vi "Check And Clear Missing Messages - XY Chart.vi"(9 "index":i32, 11 "AScan+Peaks in":cluster{"timebase":dbl[], "data":u16[]}[](array[cluster])) -> (1 "Running Average PRF":dbl, 3 "AScan+Peaks out":cluster{"timebase":dbl[], "data":u16[]}[](array[cluster]))   [LabVIEW 2026, in "MicroPulse_Driver.lvlib"]
uses:
  MicroPulse_Driver.lvlib
  <vilib>/ptbypt/NI_PtbyPt.lvlib
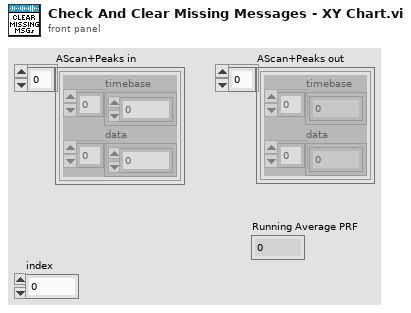
[diagram p1: front panel]
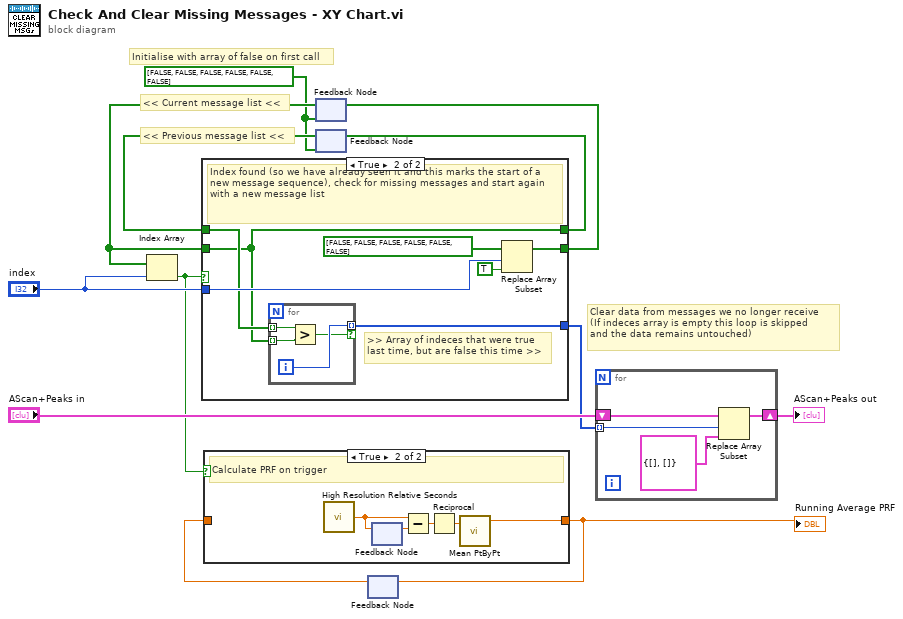
[diagram p0: block diagram]
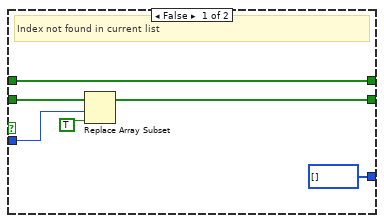
[diagram p3: hidden frame]
diagram:
  w7 = bool[] [FALSE, FALSE, FALSE, FALSE, FALSE, FALSE]
  # "Clear data from messages we no longer receive\n(If indeces array is empty this loop is skipped\nand the data remains untouched)"
  # "Initialise with array of false on first call"
  # "<< Previous message list <<"
  # "<< Current message list <<"
  n1 = feedback #1(w7) -> (w9:bool[])
  n2 = Index Array(array=w9, index="index") -> (element=w1:bool)
  n3 = feedback #2(w7) -> (w11:bool[])
  n4 = case shown="True" w1 {
    tunnel: "index" -> [w18 w23]
    tunnel: w9 -> [w17 w20]
    tunnel: [w16 w24] -> w12
    tunnel: w11 -> [w15 w21]
    tunnel: [w15 w20] -> w10
    tunnel: [i32[] [] w19] -> w5
    frame False {
      # "Index not found in current list"
      n5 = Replace Array Subset(array=w17, new element=TRUE, index=w18) -> (w16:bool[])
    }
    frame True {
      # ">> Array of indeces that were true\nlast time, but are false this time >>"
      # "Index found (so we have already seen it and this marks the start of a new message sequence), check for missing messages and start again with a new message list"
      n6 = for {
        tunnel: w21 -> [w29] mode=indexing
        tunnel: w20 -> [w28] mode=indexing
        tunnel: [w27] -> w19 mode=indexing if=w26
        i -> [w27]
        n7 = Greater?(x=w29, y=w28) -> (0:w26:bool)
      }
      n8 = Replace Array Subset(array=bool[] [FALSE, FALSE, FALSE, FALSE, FALSE, FALSE], new element=TRUE ("new element/subarray"), index=w23) -> (w24:bool[])
    }
  }
  n9 = feedback-in #1(w12) -> ()
  n10 = feedback-in #2(w10) -> ()
  n11 = feedback #3() -> (w2:dbl)  [unwired: 1 in]
  n12 = case shown="True" w1 {
    tunnel: [w30 w31] -> w3
    tunnel: w2 -> [w30 _]
    frame False {
    }
    frame True {
      # "Calculate PRF on trigger"
      n13 = call <vilib>:"High Resolution Relative Seconds.vi"() -> ("relative seconds"=w32:dbl)
      n14 = feedback #4() -> (w33:dbl)  [unwired: 1 in]
      n15 = feedback-in #4(w32) -> ()
      n16 = Subtract(x=w32, y=w33) -> (x-y=w34:dbl)
      n17 = Reciprocal(x=w34) -> (1/x=w35:dbl)
      n18 = call <vilib>:"Mean PtByPt.vi"("x"=w35) -> ("mean"=w31:dbl)  [unwired: 3 in, 1 out]
    }
  }
  "Running Average PRF" <- w3
  n19 = feedback-in #3(w3) -> ()
  n20 = for {
    shift-right: [w38] -> w4
    shift-left: "AScan+Peaks in" -> [w39]
    tunnel: w5 -> [w37] mode=indexing
    n21 = Replace Array Subset(array=w39, new element=cluster{"timebase":dbl[], "data":u16[]} {"timebase"=[], "data"=[]} ("new element/subarray"), index=w37) -> (w38:cluster{"timebase":dbl[], "data":u16[]}[])
  }
  "AScan+Peaks out" <- w4
